vi "Solinoid Control Logic.vi"(11 "Input":bool) -> (2 "Out":bool, 3 "In":bool)   [LabVIEW 2017]
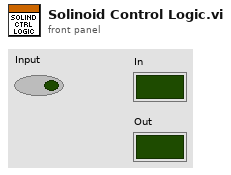
[diagram p1: front panel]
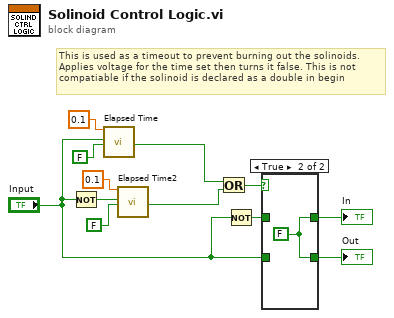
[diagram p0: block diagram]
diagram:
  # "This is used as a timeout to prevent burning out the solinoids.\nApplies voltage for the time set then turns it false. This is not\ncompatiable if the solinoid is declared as a double in begin"
  n1 = Not(x="Input") -> (.not. x?=w8:bool)
  n2 = call "Elapsed Time"("Time Target (s)"=0.1, "Reset"="Input", "Auto Reset"=FALSE) -> ("Time has Elapsed"=w7:bool)  [unwired: 9 in, 7 out]
  n3 = call "Elapsed Time2"("Time Target (s)"=0.1, "Reset"=w8, "Auto Reset"=FALSE) -> ("Time has Elapsed"=w6:bool)  [unwired: 9 in, 7 out]
  n4 = Or(x=w7, y=w6) -> (x .or. y?=w5:bool)
  n5 = Not(x="Input") -> (.not. x?=w4:bool)
  n6 = case shown="True" w5 {
    tunnel: [w14 w15] -> w10
    tunnel: [w13 w15] -> w9
    tunnel: w4 -> [w14 _]
    tunnel: "Input" -> [w13 _]
    frame False {
    }
    frame True {
      w15 = FALSE
    }
  }
  "In" <- w10
  "Out" <- w9
